vi "MathOperationSubVI.vi"(6 "Square":bool, 8 "Error In":errorcluster, 10 "Coefficient(1)":dbl=1.0, 11 "Main value in":dbl) -> (0 "Error Out":errorcluster, 3 "Result":dbl)   [LabVIEW 2020]
doc: "Simple VI with some math operation to present options of connector settings."
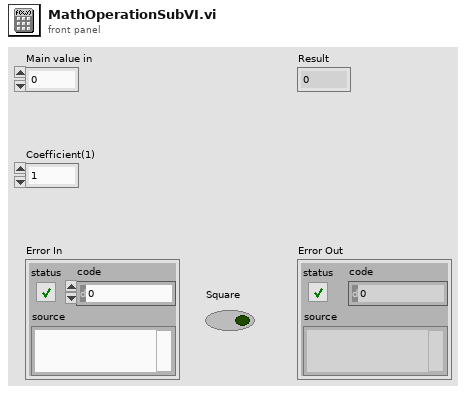
[diagram p1: front panel]
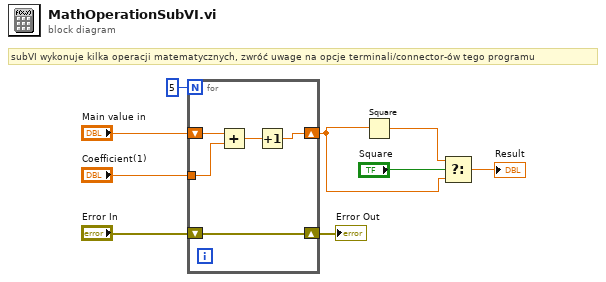
[diagram p0: block diagram]
diagram:
  # "subVI wykonuje kilka operacji matematycznych, zwróć uwage na opcje terminali/connector-ów tego programu"
  n1 = for {
    N: 5 -> [_]
    tunnel: "Coefficient(1)" -> [w13]
    shift-right: [w11] -> w3
    shift-left: "Main value in" -> [w14]
    shift-right: [w10] -> w9
    shift-left: "Error In" -> [w10]
    n2 = Add(x=w14, y=w13) -> (x+y=w12:dbl)
    n3 = Increment(x=w12) -> (x+1=w11:dbl)
  }
  "Error Out" <- w9
  n4 = Square(x=w3) -> (x^2=w2:dbl)
  n5 = Select(t=w2, s="Square", f=w3) -> (s? t:f=→"Result":dbl)
